vi "initializeProgram.vi"(10 "subpanelRef":refnum<vi>, 11 "vi folder":path) -> ()   [LabVIEW 2015]
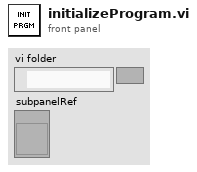
[diagram p1: front panel]
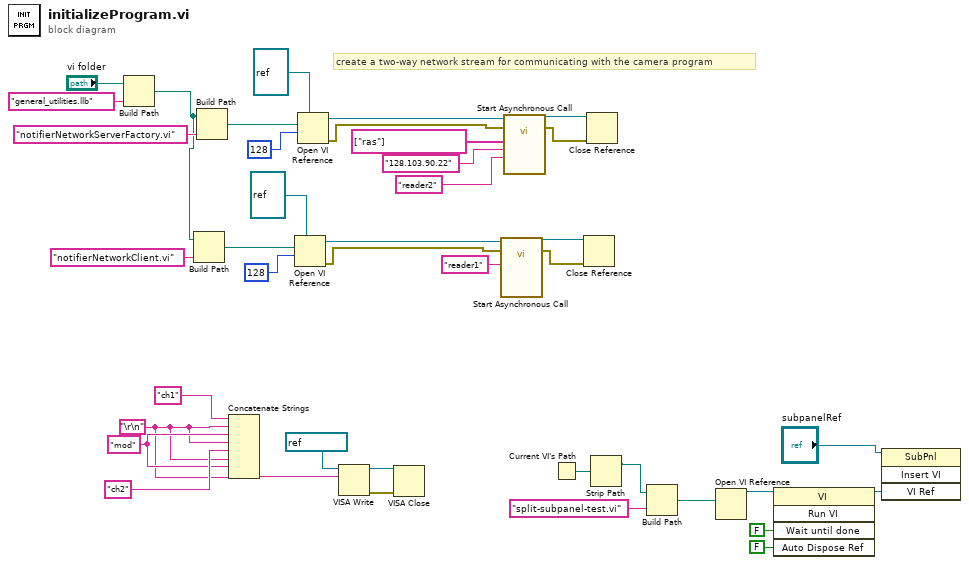
[diagram p0: block diagram]
diagram:
  w11 = "mod" ("f")
  w10 = "\r\n"
  # "create a two-way network stream for communicating with the camera program"
  n1 = Build Path(base path="vi folder", name or relative path="general_utilities.llb") -> (appended path=w19:path)
  n2 = Build Path(base path=w19, name or relative path="notifierNetworkClient.vi") -> (appended path=w25:path)
  n3 = Build Path(base path=w19, name or relative path="notifierNetworkServerFactory.vi") -> (appended path=w36:path)
  n4 = Concatenate Strings("ch1" ("string"), w10, w11, w10, "ch2" ("string"), w10, w11, w10) -> (w14:string)
  n5 = Open VI Reference(type specifier VI Refnum (for type only)=refnum<vi> refnum, vi path=w25, options=128) -> (vi reference=w26:refnum<vi>, error out=w22:errorcluster)  [unwired: 3 in]
  n6 = Open VI Reference(type specifier VI Refnum (for type only)=refnum<vi> refnum, vi path=w36, options=128) -> (vi reference=w37:refnum<vi>, error out=w30:errorcluster)  [unwired: 3 in]
  n7 = VISA Write(VISA resource name=refnum<visa-resource-name> "COM3", write buffer=w14) -> (VISA resource name out=w8:refnum<visa-resource-name>, error out=w9:errorcluster)  [unwired: 1 in, 1 out]
  n8 = VISA Close(VISA resource name=w8, error in (no error)=w9) -> ()  [unwired: 1 out]
  n9 = call-by-ref "Start Asynchronous Call"(reference=w26, error in=w22, "reader name"="reader1") -> (reference out=w24:refnum<vi>, error out=w23:errorcluster)  [unwired: 11 in]
  n10 = call-by-ref "Start Asynchronous Call"(reference=w37, error in=w30, "reader name"="reader2", "ip address"="128.103.90.22", "notifier names"=string[] ["ras"]) -> (reference out=w32:refnum<vi>, error out=w31:errorcluster)  [unwired: 9 in]
  n11 = Current VI's Path() -> (path=w16:path)
  n12 = Close Reference(reference=w24, error in (no error)=w23) -> ()  [unwired: 1 out]
  n13 = Close Reference(reference=w32, error in (no error)=w31) -> ()  [unwired: 1 out]
  n14 = Strip Path(path=w16) -> (stripped path=w1:path)  [unwired: 1 out]
  n15 = Build Path(base path=w1, name or relative path="split-subpanel-test.vi") -> (appended path=w17:path)
  n16 = Open VI Reference(vi path=w17) -> (vi reference=w4:refnum<vi>)  [unwired: 5 in, 1 out]
  n17 = invoke class="VI" method="Run VI"(reference=w4, "Wait until done"=FALSE ("Wait Until Done"), "Auto Dispose Ref"=FALSE ("Auto Dispose Reference")) -> (reference out=w3:refnum<vi>)  [unwired: 2 in, 4 out]
  n18 = invoke on="Invoke Node" class="SubPnl" method="Insert VI"(reference="subpanelRef", "VI Ref"=w3) -> ()  [unwired: 2 in, 4 out]
